vi "Edit Configrations.vi"(2 "Error In":errorcluster) -> (0 "Error Out":errorcluster)   [LabVIEW 2018]
uses:
  Type Defs/Instrument Model.ctl
  Type Defs/State Machine.ctl
  Config/Edit Config.ctl
  Type Defs/Configration.ctl
  GC-MSMSDevlopment/Type/_RT Configuration 2.ctl
  Type Defs/Global Action.ctl
  Type Defs/RT Command.ctl
  FGVs/Global Variables.vi
  <vilib>/Utility/config.llb/Read Key (Path).vi
  <vilib>/Utility/config.llb/Read Key (I32).vi
  <vilib>/Utility/config.llb/Read Key (Boolean).vi
  <vilib>/Utility/config.llb/Write Key (Path).vi
  <vilib>/Utility/config.llb/Write Key (String).vi
  <vilib>/Utility/config.llb/Write Key (Boolean).vi
  <vilib>/Utility/config.llb/Write Key (I32).vi
  <vilib>/Utility/config.llb/NI_LVConfig.lvlib
panel:
  in  "dsPIC33 4":u16
  in  "dsPIC33 3":u16
  in  "dsPIC33 2":u16
  in  "Set PIC":bool
  out "dsPIC33 Monitor":u64
  in  "dsPIC33":u16
  in  "Model Name":T1
  in  "Exit":bool
  in  "Pole Swap Options Negative":T2
  in  "Pole Swap Options Positive":T2
  in  "Dead Time":i32
  out "Number of Parameters":i32
  in  "CAD Evac T (ms)":i32
  in  "CAD Fill T (ms)":i32
  in  "S Swithc T (mS)":i32
  in  "Pole Swithc T (mS)":i32
  in  "Oscillator Settings":string[](array[string])
  in  "Restore From Power Failure":bool
  in  "Use DT Correction":bool
  in  "Enable Voltage Reset":bool
  in  "Serial Number":string
  in  "Config File Name":string
  in  "Settling Time (mS)":dbl
  in  "Description":string
  in  "Type":u8 format="%b"
  in  "Calibration Offset":dbl
  in  "Calibration Slop":dbl
  in  "User -ve Default":dbl
  in  "User +ve Default":dbl
  in  "User Maximum":dbl
  in  "User Minimum":dbl
  in  "Channel Number":u8
  in  "Parameter Name":string
  in  "Export":bool
  in  "Import":bool
  in  "Delete Row":bool
  in  "Insert Row":bool
  in  "Load":bool
  in  "Save":bool
  in  "Undo":bool
  in  "Reconnect":bool
  in  "Table":i32(listbox)
  # "Other Instrument Configrations"
  # "Pole Orientation"
  # "Current Parameters"
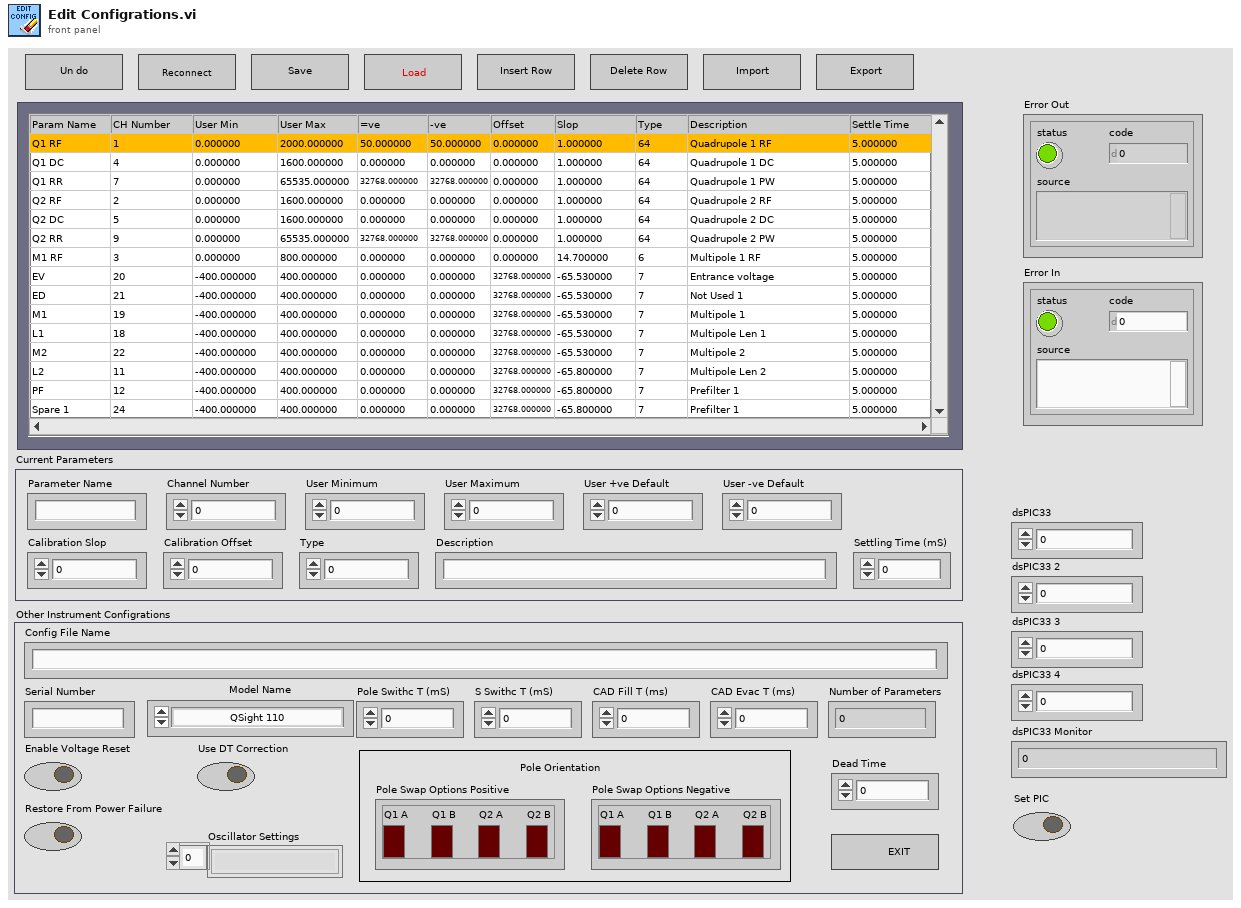
[diagram p1: front panel]
types:
  T1 = typedef "Instrument Model.ctl" = enum16{"QSight 110", "QSight 120", "QSight 210", "QSight 220", "QSight 410", "QSight 420", "IONICS 3Q 110", "IONICS 3Q 120", "IONICS 3Q 210", "IONICS 3Q 220", "IONICS 3Q 310", "IONICS 3Q 320", "Simulation (Single Source)", "Simulation (Dual Source)"}
  T2 = cluster{"Q1 A":bool, "Q1 B":bool, "Q2 A":bool, "Q2 B":bool}
  T3 = typedef "Edit Config.ctl" = cluster{"IP Address":string, "Index":i32, "Update Table":bool, "File Path":path, "Configration":T4}
  T4 = typedef "Configration.ctl" = cluster{"Table":T5[], "Instrument":string[]}
  T5 = typedef "_RT Configuration 2.ctl" = cluster{"Name":string, "Ch#":u8, "Min":dbl, "Max":dbl, "Def+":dbl, "Def-":dbl, "Offset":dbl, "Slope":dbl, "Type":u8, "Description":string, "SettleT":dbl}
  T6 = typedef "State Machine.ctl" = enum16{"Wait", "Init", "Case 0", "Case 1", "Case 2", "Case 3", "Case 4", "Case 5", "Case 6", "Case 7", "Case 8", "Case 9", "Case 10", "Error", "Exit"}
  T7 = typedef "Global Action.ctl" = enum16{"Write", "Read"}
  T8 = typedef "RT Command.ctl" = enum16{"xml Start Run", "xml Start Actual Run", "xml Stop Run", "xml Runtime Update", "xml Get Status", "xml Get Table", "xml Set Table", "xml Get Configuration", "xml System Status", "xml Set LC Input Logic", "xml Get Data", "xml Get Info", "Start", "StartActualRun", "Stop", "Runtime Update", "Get Data", "Get Info", "Get Status", "Get Param", "Get Config", "Get Table", "Read ADC", "Set Oscillator", "Update Config", "Update Table", "Set All Pol", "Set Pol and DC", "Set Max Mass", "Toggle RP", "Toggle EL", "Set PIC", "Initialize Turbo", "Send Turbo Comm", "Close Turbo", "P1", "P2", "P3", "Send Serial", "Set LC Out", "Get LC In", "Read VAC", "Test Table", "Toggle Power", "Get Startup", "Set Startup", "Get ADC Table", "Set ADC Table", "Get Brief Status", "Get Detail Status", "Auxiliary Update", "Set CC Logics", "Set CC Input Logics", "Ignore Error", "invalid"}
  T9 = typedef "Global Configrations.ctl" = cluster{"Model Name":enum16{"QSight 110", "QSight 120", "QSight 210", "QSight 220", "QSight 410", "QSight 420", "IONICS 3Q 110", "IONICS 3Q 120", "IONICS 3Q 210", "IONICS 3Q 220", "IONICS 3Q 310", "IONICS 3Q 320", "Simulation (Single Source)", "Simulation (Dual Source)"}, "RunType":u16, "Acquisition State":enum16{"Ready", "Busy", "Waiting"}, "InstrState":enum16{"Initializing", "Mass Spectrometer is Off", "Starting Up", "Turning Power Off", "Going to Standby", "Roughing Pump Ready", "Turning Turbo Off", "Turbo Startup", "Turbopump Ready", "Checking Vacuum", "Going to Ready", "Ready", "Running", "Source Standby", "Lost Communication", "Shutting Down", "Fault", "24V Standby", "Go to 24V Standby", "Turbopump Ready-Waiting"}, "Run Mode":enum16{"MRM (Q1/Q2)", "Q1 Scan", "Q1 SRM", "Q2 Scan", "Q2 SRM", "Product Scan", "Precursor Scan", "Neutral Loss", "Neutral Gain"}, "Configration":T4, "TCP ID":refnum<k5>, "DT":bool, "Dead Time (nS)":i32, "Single Source":bool, "ADC Tables":T10[], "FW Udate":bool, "Simulator":bool}
  T10 = typedef "ADC Table.ctl" = cluster{"Name":string, "Ch#":u8, "Min":dbl, "Max":dbl, "Def+":dbl, "Def-":dbl, "Offset":dbl, "Slope":dbl, "Type":u8, "Description":string, "SettleT":dbl}
  T11 = typedef "NI_LVConfig.lvlib/Config Data RefNum.ctl" = refnum<k1>
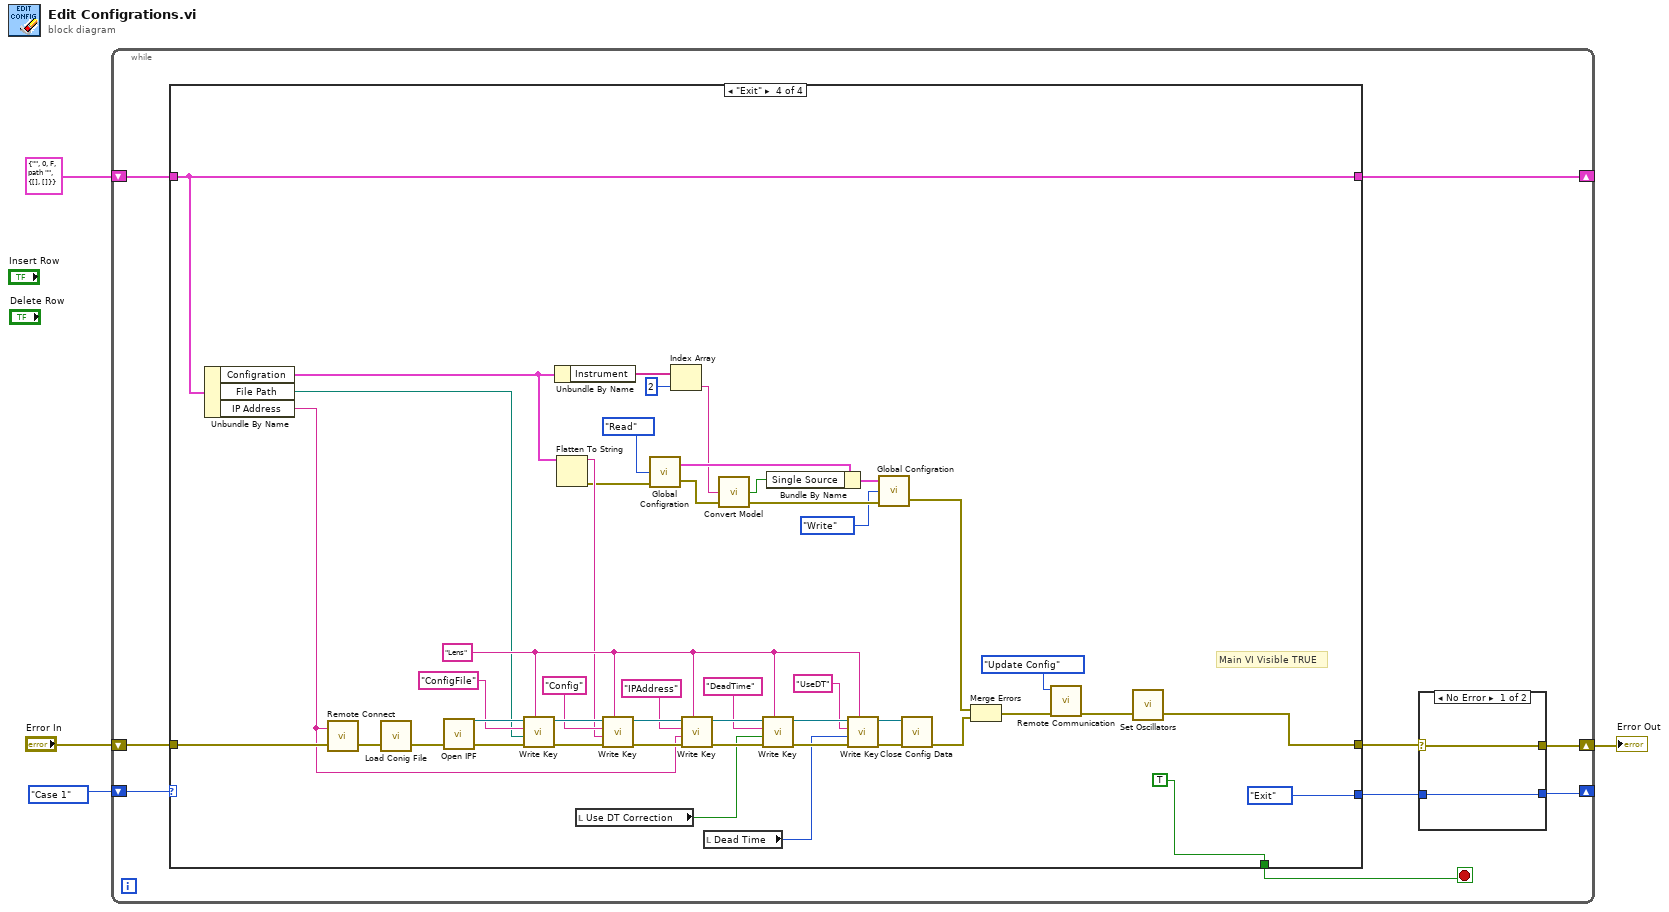
[diagram p0: block diagram]
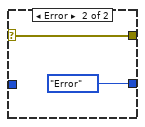
[diagram p2: hidden frame]
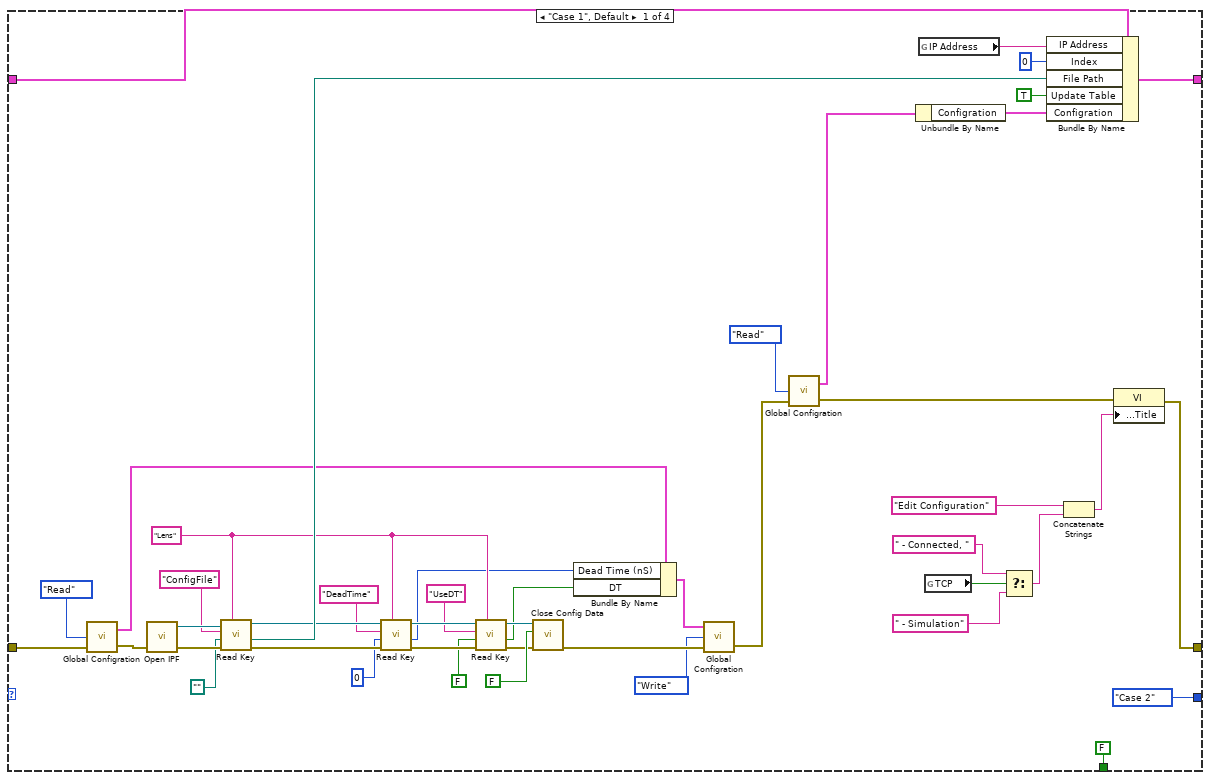
[diagram p3: hidden frame]
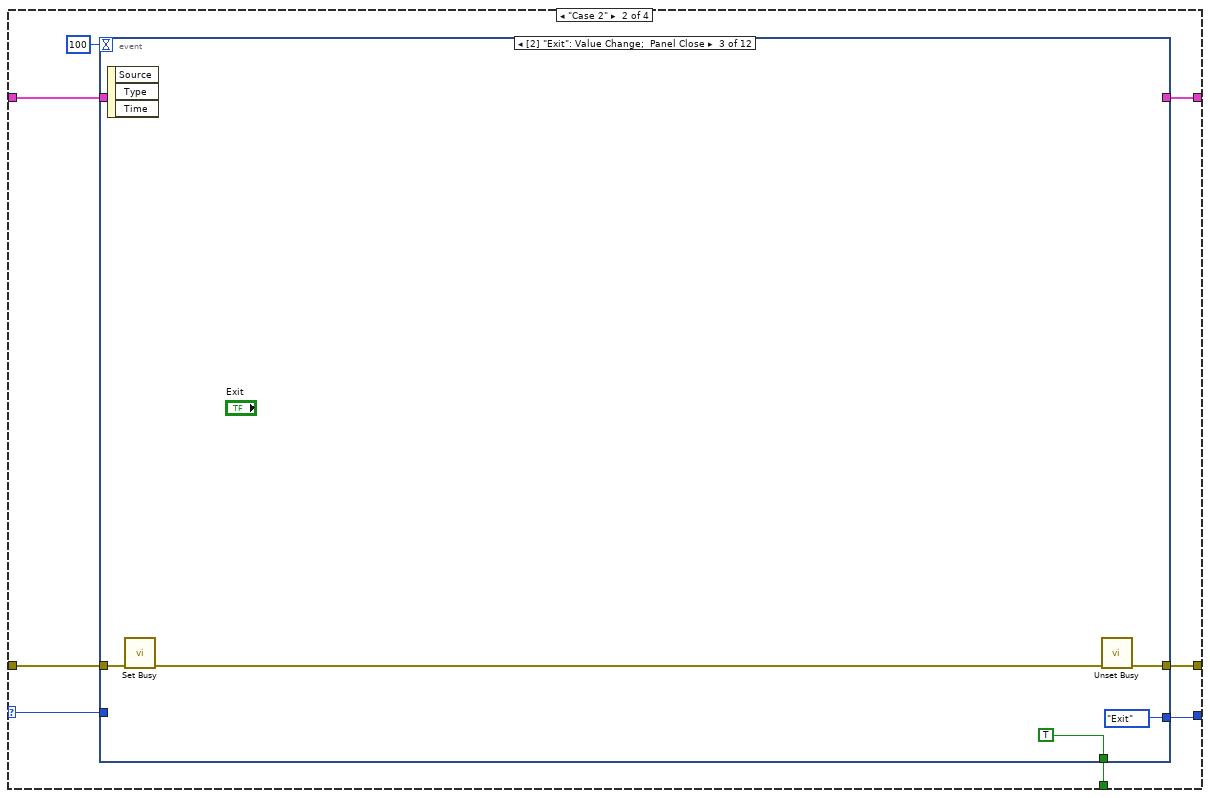
[diagram p4: hidden frame]
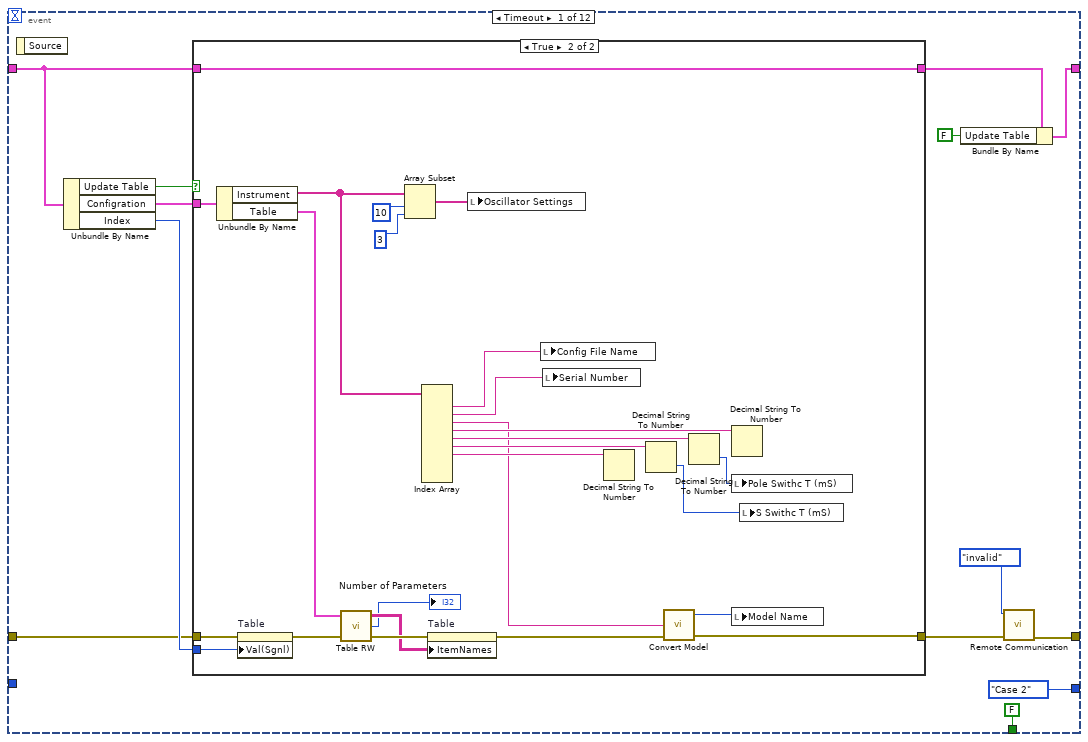
[diagram p5: hidden frame]
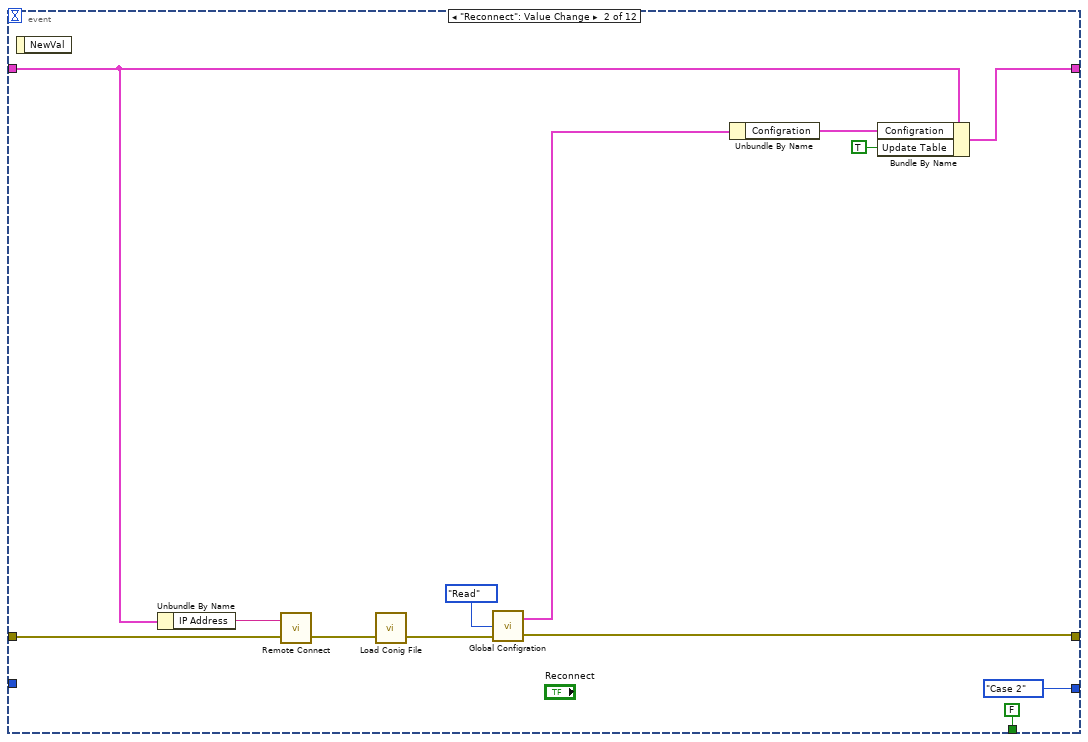
[diagram p7: hidden frame]
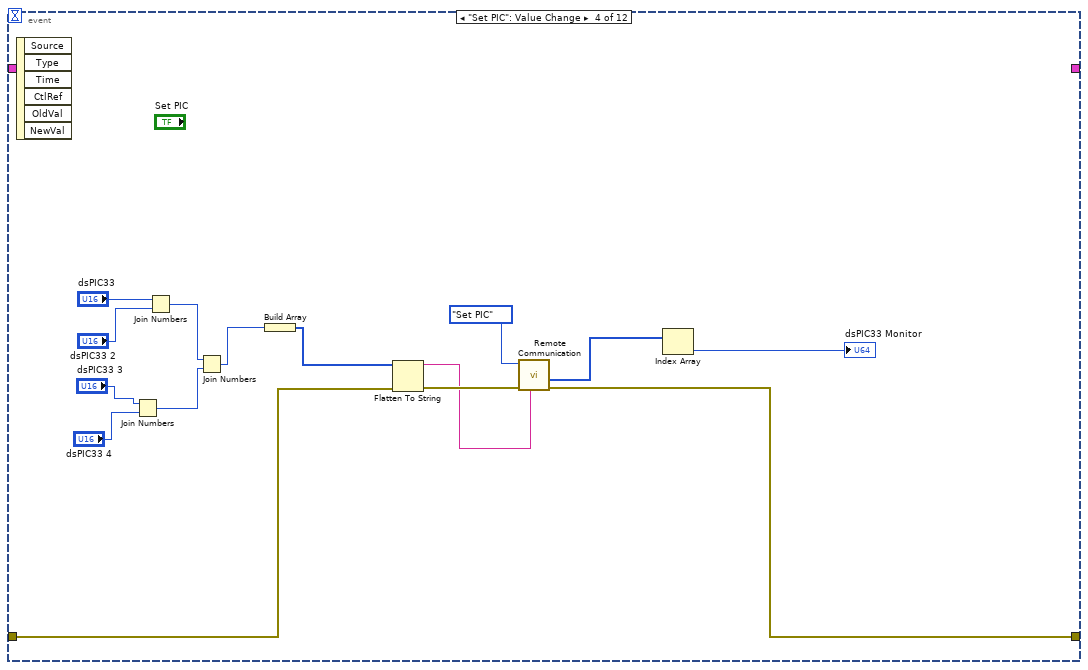
[diagram p8: hidden frame]
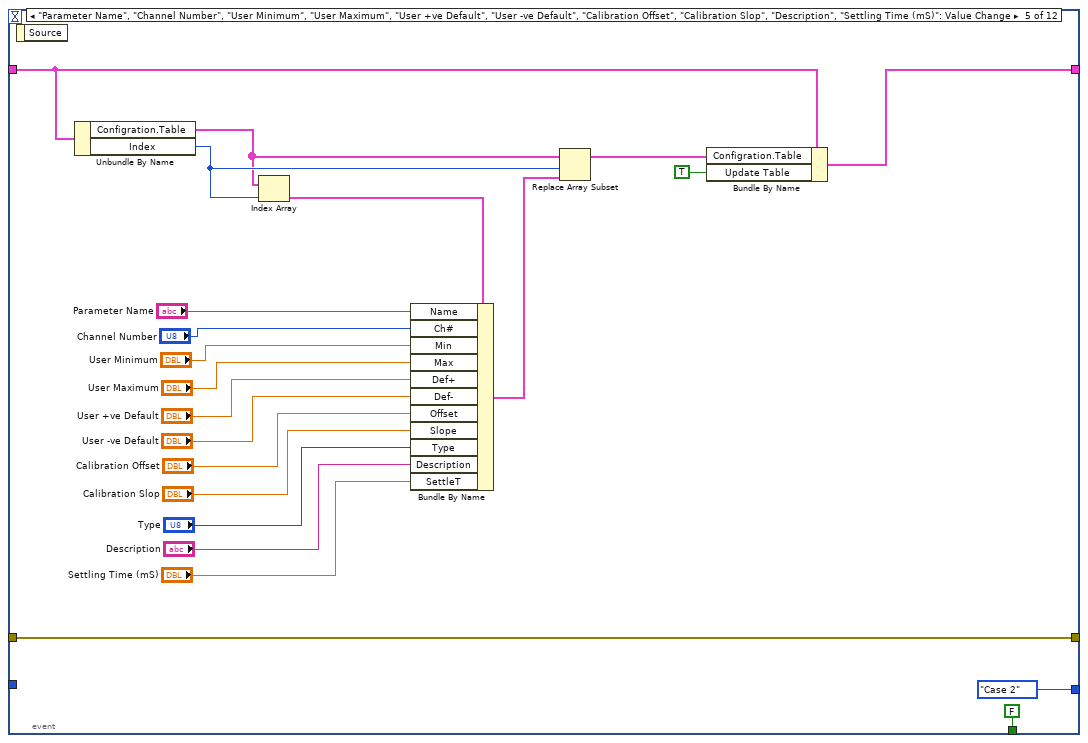
[diagram p9: hidden frame]
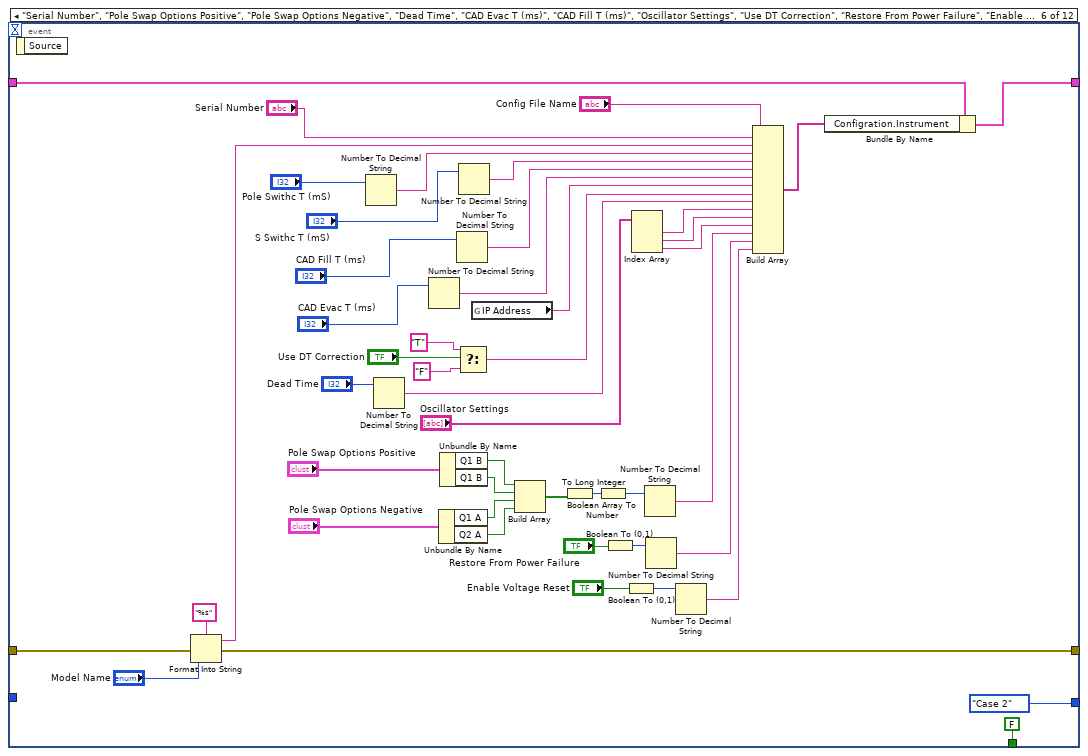
[diagram p10: hidden frame]
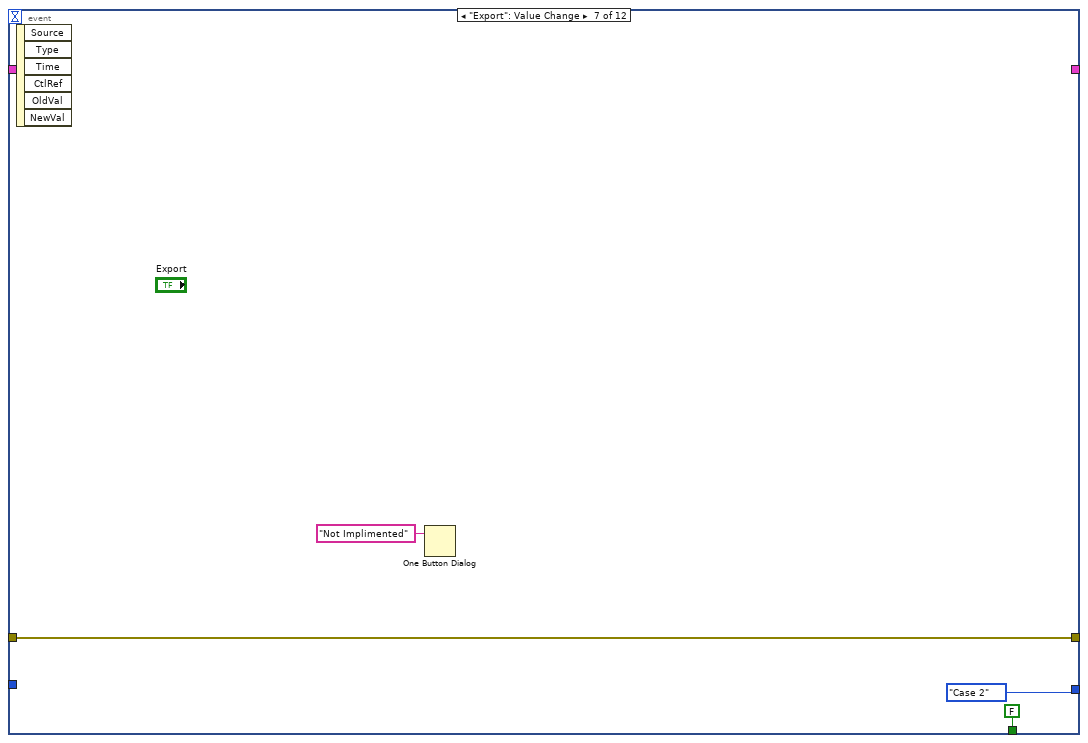
[diagram p11: hidden frame]
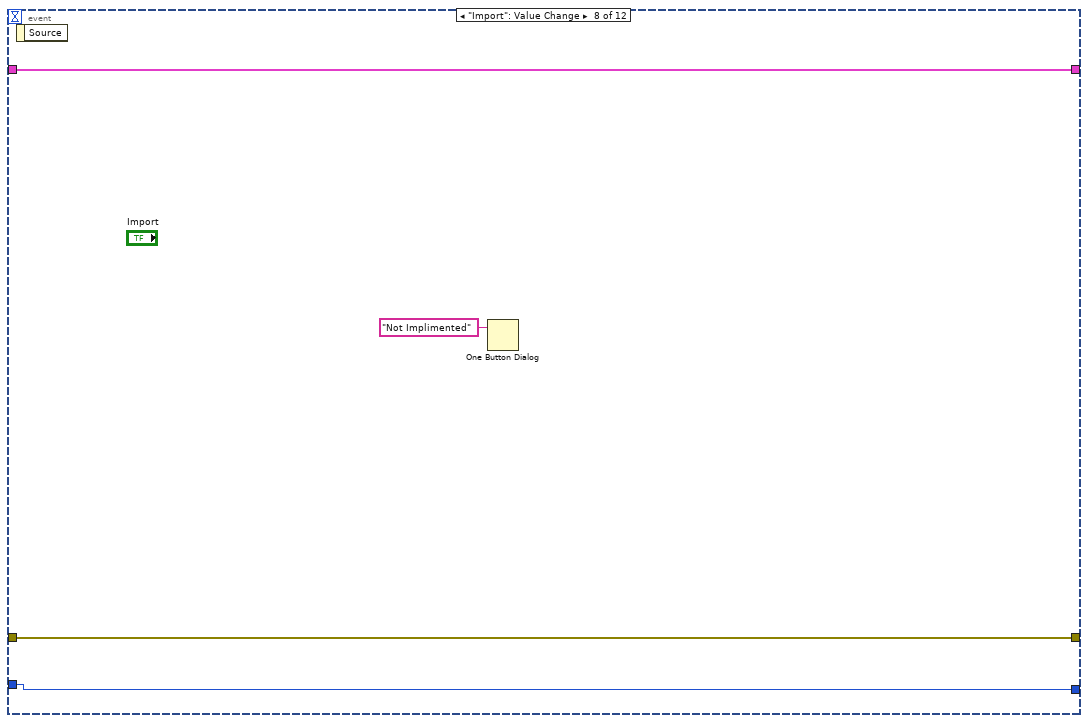
[diagram p12: hidden frame]
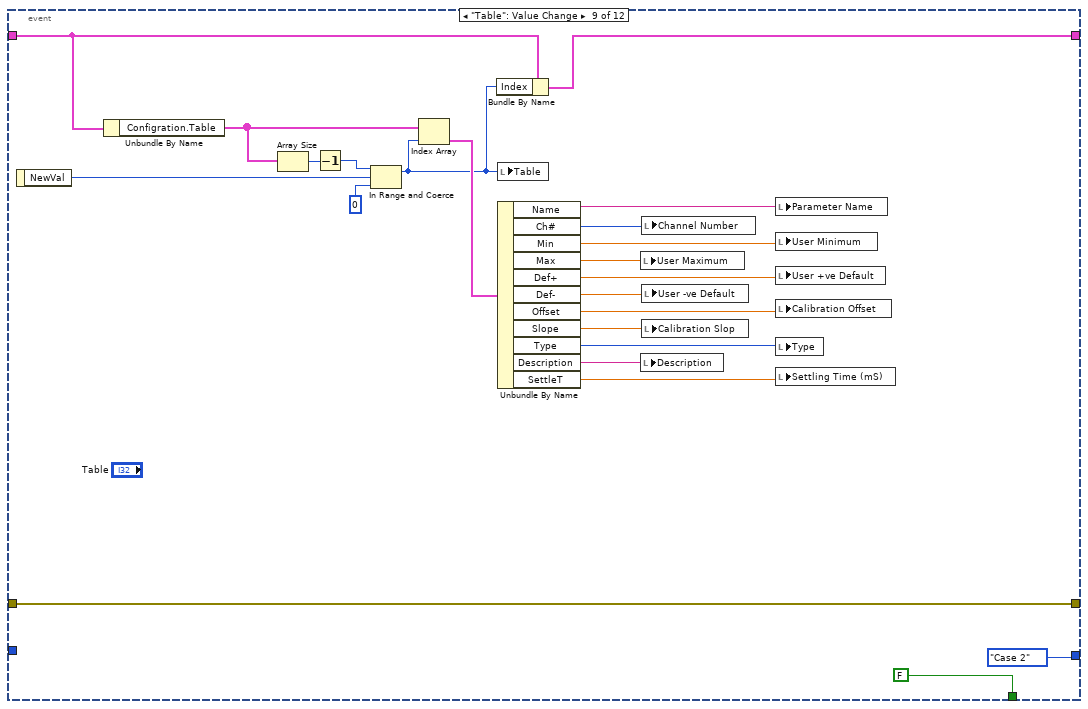
[diagram p13: hidden frame]
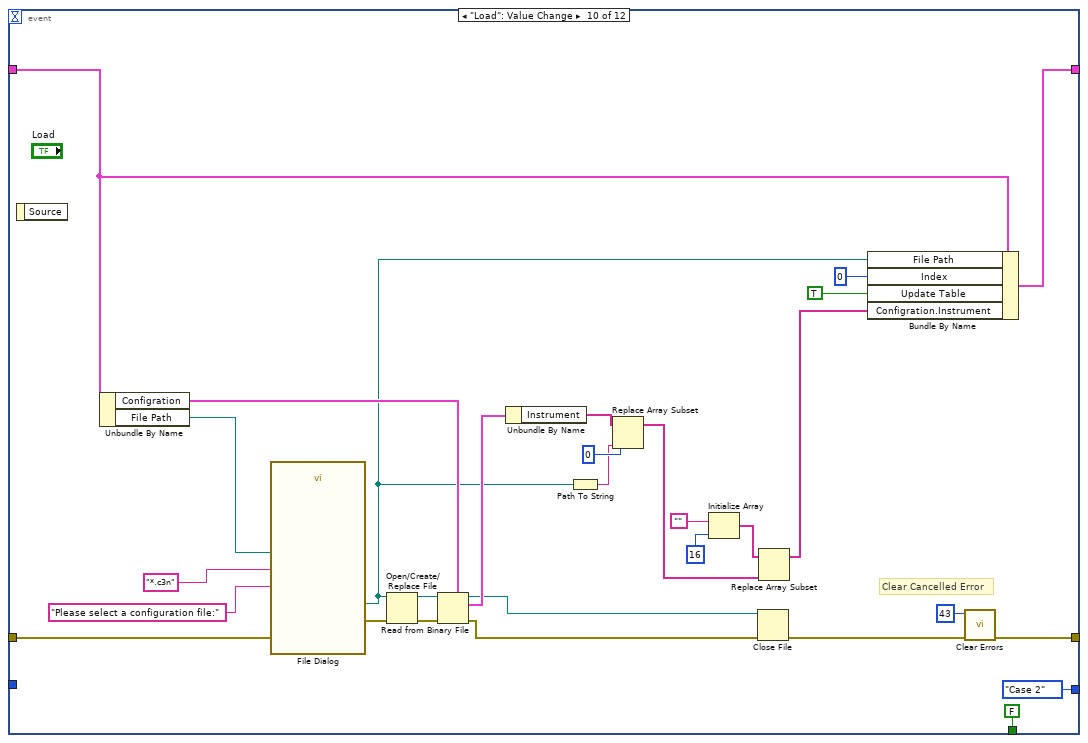
[diagram p14: hidden frame]
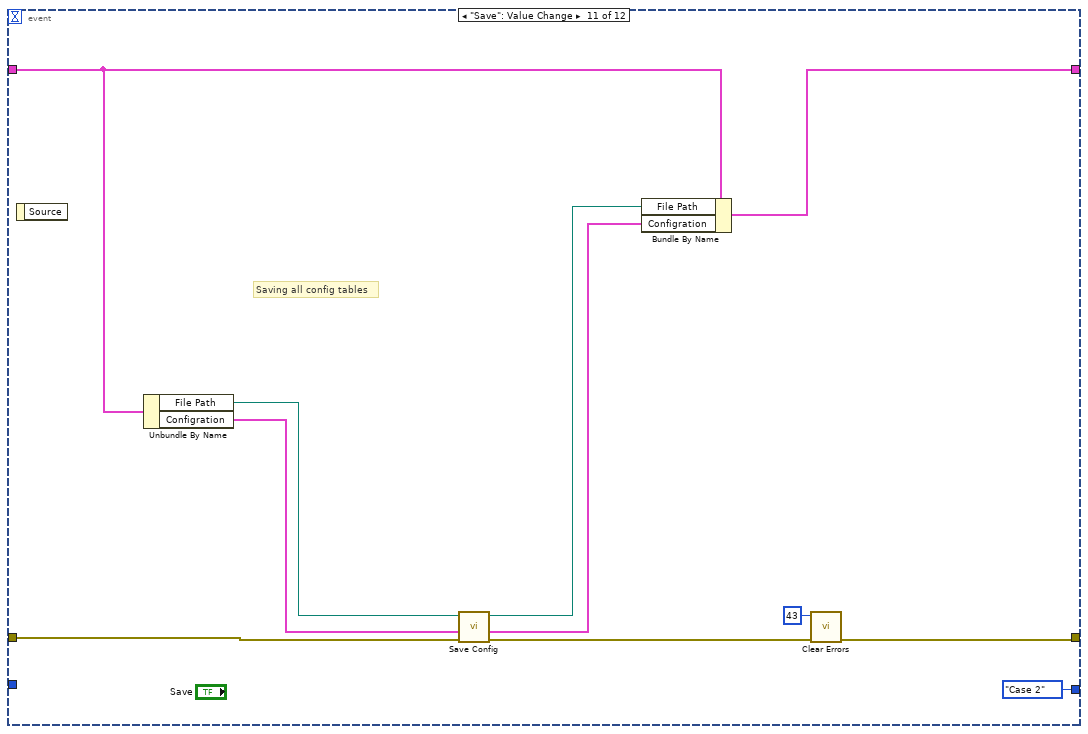
[diagram p15: hidden frame]
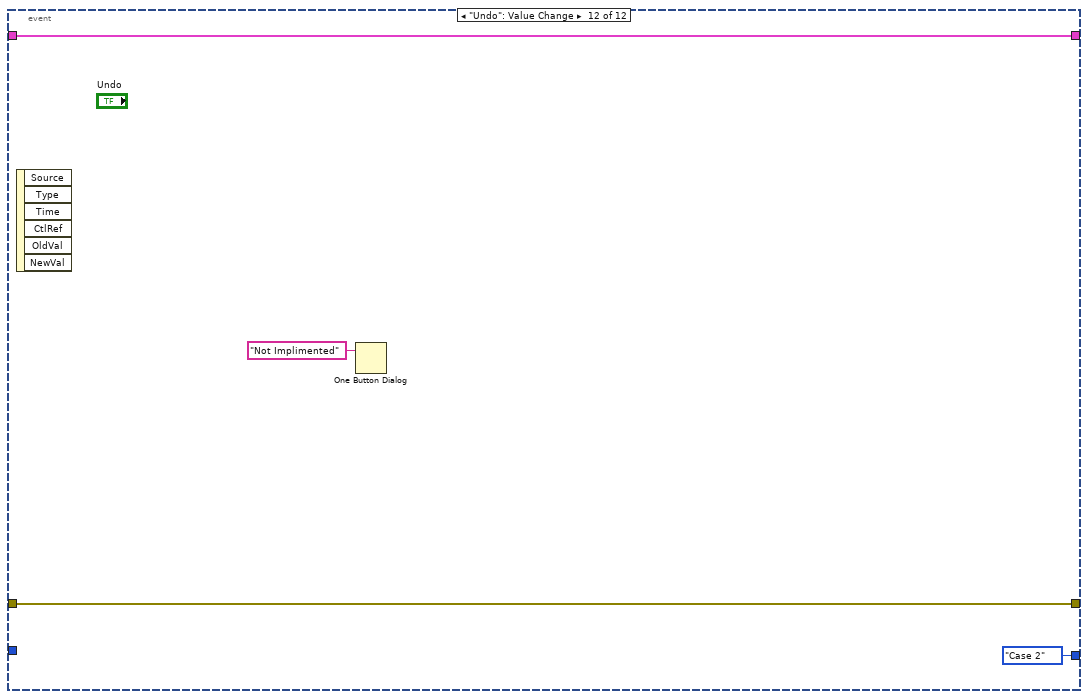
[diagram p16: hidden frame]
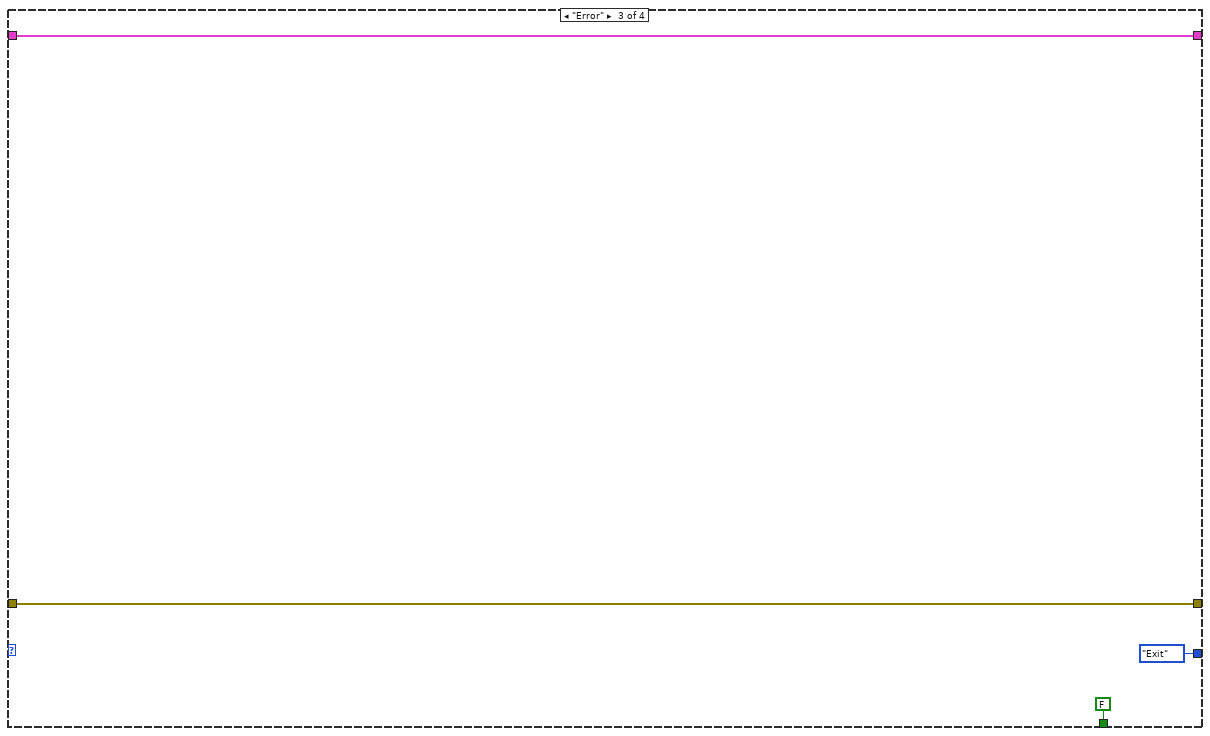
[diagram p17: hidden frame]
diagram:
  n1 = while {
    shift-right: [w8] -> _
    shift-left: State_Machine."Case 1" -> [w13]
    shift-right: [w11] -> _
    shift-left: T3 {"IP Address"="", "Index"=0, "Update Table"=FALSE, "File Path"=path "", "Configration"={"Table"=[], "Instrument"=[]}} ("Edit Configrations") -> [w10]
    shift-right: [w6] -> w2
    shift-left: "Error In" -> [w12]
    stop <- w5 stop-if-true
    n2 = case shown="\"Exit\"" w13 {
      selector: w13 -> [_ w66 _ _]
      tunnel: w12 -> [w27 w69 w288 w313]
      tunnel: [w62 w67 w289 w337] -> w11
      tunnel: [w50 w68 w288 w292] -> w9
      tunnel: w10 -> [w24 w70 w289 w337]
      tunnel: [State_Machine."Case 2" w64 State_Machine."Exit" State_Machine."Exit"] -> w7
      tunnel: [FALSE w63 FALSE TRUE] -> w5
      frame "Case 1", Default {
        w40 = "Lens" ("section")
        n3 = call "Global Configration.vi"("Error In"=w27, "Action"=Global_Action."Read") -> ("Error Out"=w28:errorcluster, "Parameters Out"=w25:T9)  [unwired: 1 in]
        n4 = call "Open IPF.vi"("Error In"=w28) -> ("Error Out"=w57:errorcluster, "IPF refnum"=w56:T11)  [unwired: 2 in, 1 out]
        n5 = call-poly <vilib>:"Read Key.vi"("section"=w40, "error in (no error)"=w57, "default value"=path "", "key"="ConfigFile", "refnum"=w56) -> ("error out"=w52:errorcluster, "value"=w53:path, "refnum out"=w51:T11)  [unwired: 4 out]
        n6 = call-poly <vilib>:"Read Key.vi"("section"=w40, "error in (no error)"=w52, "default value"=0, "key"="DeadTime", "refnum"=w51) -> ("error out"=w43:errorcluster, "value"=w31:i32, "refnum out"=w41:T11)  [unwired: 4 out]
        n7 = call-poly <vilib>:"Read Key.vi"("section"=w40, "error in (no error)"=w43, "default value"=FALSE, "key"="UseDT", "refnum"=w41) -> ("error out"=w34:errorcluster, "value"=w32:bool, "refnum out"=w42:T11)  [unwired: 4 out]
        n8 = call <vilib>:"Close Config Data.vi"("error in (no error)"=w34, "write file if changed (T)"=FALSE, "refnum"=w42) -> ("error out"=w30:errorcluster)  [unwired: 8 out]
        n9 = Bundle By Name(cluster=w25, "Dead Time (nS)"=w31, "DT"=w32) -> (w33:T9)
        n10 = call "Global Configration.vi"("Error In"=w30, "Action"=Global_Action."Write", "Parameters In"=w33) -> ("Error Out"=w20:errorcluster)  [unwired: 1 out]
        n11 = call "Global Configration.vi"("Error In"=w20, "Action"=Global_Action."Read") -> ("Error Out"=w21:errorcluster, "Parameters Out"=w19:T9)  [unwired: 1 in]
        n12 = Unbundle By Name(w19) -> ("Configration"=w58:T4)
        n13 = global read "Global Variables.vi" "IP Address"() -> (w61:string)
        n14 = global read "Global Variables.vi" "TCP"() -> (w46:bool)
        n15 = Select(t=" - Connected, " ("string"), s=w46, f=" - Simulation" ("string")) -> (s? t:f=w47:string)
        n16 = Bundle By Name(cluster=w24, "IP Address"=w61, "Index"=0, "File Path"=w53, "Update Table"=TRUE, "Configration"=w58) -> (w62:T3)
        n17 = Concatenate Strings("Edit Configuration" ("string"), w47) -> (w44:string)
        n18 = property class="VI"(error in=w21, "Front Panel Window:Title"=w44) -> (error out=w50:errorcluster)  [unwired: 1 in, 1 out]
      }
      frame "Case 2" {
        n19 = event shown="[2] \"Exit\": Value Change;  Panel Close" {
          selector: _ -> [_ _ _ _ _ _ _ _ _ _ _ _]
          dyn-events: _ -> [_ _ _ _ _ _ _ _ _ _ _ _]
          timeout: 100 -> [_ _ _ _ _ _ _ _ _ _ _ _]
          tunnel: w70 -> [w76 w119 _ _ w161 w212 _ w219 w235 w263 w280 w286]
          tunnel: [FALSE FALSE TRUE _ FALSE FALSE FALSE _ FALSE FALSE _ _] -> w63
          tunnel: w69 -> [w78 w123 w126 w141 w146 w205 w215 w218 w242 w270 w283 w285]
          tunnel: [w73 w113 w125 w138 w146 w203 w215 w218 w242 w244 w274 w285] -> w68
          tunnel: [w83 w118 _ _ w158 w211 _ w219 w234 w249 w277 w286] -> w67
          tunnel: w66 -> [_ _ _ _ _ _ _ w217 _ _ _ _]
          tunnel: [State_Machine."Case 2" State_Machine."Case 2" State_Machine."Exit" _ State_Machine."Case 2" State_Machine."Case 2" State_Machine."Case 2" w217 State_Machine."Case 2" State_Machine."Case 2" State_Machine."Case 2" State_Machine."Case 2"] -> w64
          event Timeout {
            n20 = event-data() -> ()  [unwired: 1 in, 1 out]
            n21 = Unbundle By Name(w76) -> ("Update Table"=w81:bool, "Configration"=w80:T4, "Index"=w79:i32)
            n22 = case shown="True" w81 {
              tunnel: w80 -> [_ w110]
              tunnel: w79 -> [_ w108]
              tunnel: w78 -> [w85 w109]
              tunnel: [w85 w90] -> w72
              tunnel: [w84 w86] -> w75
              tunnel: w76 -> [w84 w86]
              frame False {
              }
              frame True {
                n23 = Unbundle By Name(w110) -> ("Instrument"=w88:string[], "Table"=w106:T5[])
                n24 = property on="Table" class="MCListbox (strict)"(error in=w109, "Val(Sgnl)"=w108) -> (error out=w107:errorcluster)  [unwired: 1 in, 1 out]
                n25 = call "Table RW.vi"("Error In"=w107, "Table In"=w106) -> ("Error Out"=w105:errorcluster, "Number of param"=→"Number of Parameters":i32, "List Out"=w104:string[][])  [unwired: 1 in]
                n26 = Array Subset(array=w88, index=10, length=3) -> (w99:string[])
                n27 = Index Array(array=w88) -> (element #1=w103:string, element #2=w102:string, element #3=w89:string, element #4=w98:string, element #5=w97:string, element #6=w96:string, element #7=w95:string)  [unwired: 10 in, 3 out]
                n28 = property on="Table" class="MCListbox (strict)"(error in=w105, "ItemNames"=w104) -> (error out=w91:errorcluster)  [unwired: 1 in, 1 out]
                n29 = local write "Oscillator Settings"(w99) -> ()
                n30 = local write "Config File Name"(w103) -> ()
                n31 = local write "Serial Number"(w102) -> ()
                n32 = Decimal String To Number(string=w95) -> ()  [unwired: 4 out]
                n33 = Decimal String To Number(string=w96) -> (number=w93:i32)  [unwired: 3 out]
                n34 = call "Convert Model.vi"("error in (no error)"=w91, "Model"=w89) -> ("error out"=w90:errorcluster, "Model Name  Out"=w87:T1)  [unwired: 1 in, 1 out]
                n35 = Decimal String To Number(string=w97) -> (number=w94:i32)  [unwired: 3 out]
                n36 = Decimal String To Number(string=w98) -> ()  [unwired: 4 out]
                n37 = local write "Pole Swithc T (mS)"(w94) -> ()
                n38 = local write "Model Name"(w87) -> ()
                n39 = local write "S Swithc T (mS)"(w93) -> ()
              }
            }
            n40 = Bundle By Name(cluster=w75, "Update Table"=FALSE) -> (w83:T3)
            n41 = call "Remote Communication.vi"("Error In"=w72, "Command"=RT_Command."invalid") -> ("Error Out"=w73:errorcluster)  [unwired: 4 in, 3 out]
          }
          event "Reconnect": Value Change {
            n42 = event-data() -> ()  [unwired: 1 in, 1 out]
            n43 = Unbundle By Name(w119) -> ("IP Address"=w122:string)
            n44 = call "Remote Connect.vi"("Error In"=w123, "IP Address"=w122) -> ("Error Out"=w121:errorcluster)  [unwired: 1 out]
            n45 = call "Load Conig File.vi"("error in (no error)"=w121) -> ("error out"=w117:errorcluster)  [unwired: 1 in, 1 out]
            n46 = call "Global Configration.vi"("Error In"=w117, "Action"=Global_Action."Read") -> ("Error Out"=w113:errorcluster, "Parameters Out"=w115:T9)  [unwired: 1 in]
            n47 = Unbundle By Name(w115) -> ("Configration"=w114:T4)
            n48 = Bundle By Name(cluster=w119, "Configration"=w114, "Update Table"=TRUE) -> (w118:T3)
          }
          event "Exit": Value Change; Panel Close {
            n49 = event-data() -> ()  [unwired: 1 in, 3 out]
            n50 = call <vilib>:"Set Busy.vi"("error in (no error)"=w126) -> ("error out"=w124:errorcluster)  [unwired: 9 in, 1 out]
            n51 = call <vilib>:"Unset Busy.vi"("error in (no error)"=w124) -> ("error out"=w125:errorcluster)  [unwired: 10 in]
          }
          event "Set PIC": Value Change {
            n52 = event-data() -> ()  [unwired: 1 in, 6 out]
            n53 = Join Numbers(hi="dsPIC33 3", lo="dsPIC33 4") -> ((hi.lo)=w129:u32)
            n54 = Join Numbers(hi="dsPIC33", lo="dsPIC33 2") -> ((hi.lo)=w130:u32)
            n55 = Join Numbers(hi=w130, lo=w129) -> ((hi.lo)=w131:u64)
            n56 = Build Array(w131) -> (w142:u64[])
            n57 = Flatten To String(anything=w142, error in (no error)=w141) -> (data string=w140:string, error out=w143:errorcluster)  [unwired: 3 out]
            n58 = call "Remote Communication.vi"("String"=w140, "Error In"=w143, "Command"=RT_Command."Set PIC") -> ("Error Out"=w138:errorcluster, "Data Array"=w134:i32[])  [unwired: 3 in, 2 out]
            n59 = Index Array(array=w134) -> (element=→"dsPIC33 Monitor":i32)  [unwired: 1 in]
          }
          event "Parameter Name", "Channel Number", "User Minimum", "User Maximum", "User +ve Default", "User -ve Default", "Calibration Offset", "Calibration Slop", "Description", "Settling Time (mS)": Value Change {
            n60 = event-data() -> ()  [unwired: 1 in, 1 out]
            n61 = Unbundle By Name(w161) -> ("Configration.Table"=w163:T5[], "Index"=w164:i32)
            n62 = Index Array(array=w163, index=w164) -> (element=w165:T5)
            n63 = Bundle By Name(cluster=w165, "Name"="Parameter Name", "Ch#"="Channel Number", "Min"="User Minimum", "Max"="User Maximum", "Def+"="User +ve Default", "Def-"="User -ve Default", "Offset"="Calibration Offset", "Slope"="Calibration Slop", "Type"="Type", "Description"="Description", "SettleT"="Settling Time (mS)") -> (w162:T5)
            n64 = Replace Array Subset(array=w163, new element=w162, index=w164) -> (w160:T5[])
            n65 = Bundle By Name(cluster=w161, "Configration.Table"=w160, "Update Table"=TRUE) -> (w158:T3)
          }
          event "Serial Number", "Pole Swap Options Positive", "Pole Swap Options Negative", "Dead Time", "CAD Evac T (ms)", "CAD Fill T (ms)", "Oscillator Settings", "Use DT Correction", "Restore From Power Failure", "Enable Voltage Reset": Value Change {
            n66 = event-data() -> ()  [unwired: 1 in, 1 out]
            n67 = Format Into String(format string="%s", error in=w205, "Model Name") -> (resulting string=w204:string, error out=w203:errorcluster)  [unwired: 1 in]
            n68 = Number To Decimal String(number="Pole Swithc T (mS)") -> (decimal integer string=w201:string)  [unwired: 1 out]
            n69 = Number To Decimal String(number="Dead Time") -> (decimal integer string=w188:string)  [unwired: 1 out]
            n70 = Number To Decimal String(number="CAD Evac T (ms)") -> (decimal integer string=w197:string)  [unwired: 1 out]
            n71 = Unbundle By Name("Pole Swap Options Negative") -> ("Q1 A"=w183:bool, "Q2 A"=w182:bool)
            n72 = Unbundle By Name("Pole Swap Options Positive") -> ("Q1 B"=w185:bool, "Q1 B"=w184:bool)
            n73 = Number To Decimal String(number="CAD Fill T (ms)") -> (decimal integer string=w198:string)  [unwired: 1 out]
            n74 = Select(t="T", s="Use DT Correction", f="F") -> (s? t:f=w192:string)
            n75 = Number To Decimal String(number="S Swithc T (mS)") -> (decimal integer string=w199:string)  [unwired: 1 out]
            n76 = global read "Global Variables.vi" "IP Address"() -> (w194:string)
            n77 = Build Array(w185, w184, w183, w182) -> (w179:bool[])
            n78 = Boolean Array To Number(Boolean array=w179) -> (number=w181:u32)
            n79 = To Long Integer(number=w181) -> (32bit integer=w180:i32)
            n80 = Boolean To (0,1)(Boolean="Restore From Power Failure") -> (0, 1=w172:i16)
            n81 = Boolean To (0,1)(Boolean="Enable Voltage Reset") -> (0, 1=w170:i16)
            n82 = Index Array(array="Oscillator Settings") -> (element #1=w177:string, element #2=w176:string, element #3=w175:string)  [unwired: 3 in]
            n83 = Number To Decimal String(number=w180) -> (decimal integer string=w174:string)  [unwired: 1 out]
            n84 = Number To Decimal String(number=w172) -> (decimal integer string=w169:string)  [unwired: 1 out]
            n85 = Number To Decimal String(number=w170) -> (decimal integer string=w168:string)  [unwired: 1 out]
            n86 = Build Array("Config File Name", "Serial Number", w204, w201, w199, w198, w197, w194, w192, w188, w177, w176, w175, w174, w169, w168) -> (w210:string[])
            n87 = Bundle By Name(cluster=w212, "Configration.Instrument"=w210) -> (w211:T3)
          }
          event "Export": Value Change {
            n88 = event-data() -> ()  [unwired: 1 in, 6 out]
            n89 = One Button Dialog(message="Not Implimented") -> ()  [unwired: 1 in, 1 out]
          }
          event "Import": Value Change {
            n90 = event-data() -> ()  [unwired: 1 in, 1 out]
            n91 = One Button Dialog(message="Not Implimented") -> ()  [unwired: 1 in, 1 out]
          }
          event "Table": Value Change {
            n92 = event-data() -> ("NewVal"=w236:i32)  [unwired: 1 in]
            n93 = Unbundle By Name(w235) -> ("Configration.Table"=w237:T5[])
            n94 = Array Size(array=w237) -> (size(s)=w240:i32)
            n95 = Decrement(x=w240) -> (x-1=w238:i32)
            n96 = In Range and Coerce(upper limit=w238, x=w236, lower limit=0) -> (coerced(x)=w233:i32)  [unwired: 1 out]
            n97 = Index Array(array=w237, index=w233) -> (element=w241:T5)
            n98 = Bundle By Name(cluster=w235, "Index"=w233) -> (w234:T3)
            n99 = local write "Table"(w233) -> ()
            n100 = Unbundle By Name(w241) -> ("Name"=w226:string, "Ch#"=w230:u8, "Min"=w224:dbl, "Max"=w225:dbl, "Def+"=w223:dbl, "Def-"=w222:dbl, "Offset"=w221:dbl, "Slope"=w227:dbl, "Type"=w228:u8, "Description"=w232:string, "SettleT"=w229:dbl)
            n101 = local write "User Maximum"(w225) -> ()
            n102 = local write "Description"(w232) -> ()
            n103 = local write "Channel Number"(w230) -> ()
            n104 = local write "User -ve Default"(w222) -> ()
            n105 = local write "Calibration Slop"(w227) -> ()
            n106 = local write "Parameter Name"(w226) -> ()
            n107 = local write "User Minimum"(w224) -> ()
            n108 = local write "User +ve Default"(w223) -> ()
            n109 = local write "Calibration Offset"(w221) -> ()
            n110 = local write "Type"(w228) -> ()
            n111 = local write "Settling Time (mS)"(w229) -> ()
          }
          event "Load": Value Change {
            # "Clear Cancelled Error"
            n112 = event-data() -> ()  [unwired: 1 in, 1 out]
            n113 = Unbundle By Name(w263) -> ("Configration"=w262:T4, "File Path"=w267:path)
            n114 = call "File Dialog"("start path"=w267, "prompt"="Please select a configuration file:", "error in"=w270, "pattern (all files)"="*.c3n" ("pattern (*.cfg)")) -> ("selected path"=w253:path, "error out"=w266:errorcluster)  [unwired: 8 in, 2 out]
            n115 = Open/Create/Replace File(file path (use dialog)=w253, error in=w266) -> (refnum out=w264:refnum<file>, error out=w265:errorcluster)  [unwired: 4 in, 1 out]
            n116 = Read from Binary File(5:w262, 8:w265, 11:w264) -> (0:w248:errorcluster, 2:w254:T4, 3:w247:refnum<file>)  [unwired: 4 out]
            n117 = Unbundle By Name(w254) -> ("Instrument"=w261:string[])
            n118 = Path To String(path=w253) -> (string=w259:string)
            n119 = Replace Array Subset(array=w261, new element=w259, index=0) -> (w255:string[])
            n120 = Initialize Array("", 16 ("dimension size")) -> (w258:string[])
            n121 = Close File(refnum=w247, error in=w248) -> (error out=w245:errorcluster)  [unwired: 1 out]
            n122 = Replace Array Subset(array=w258, new element=w255) -> (w250:string[])  [unwired: 1 in]
            n123 = Bundle By Name(cluster=w263, "File Path"=w253, "Index"=0, "Update Table"=TRUE, "Configration.Instrument"=w250) -> (w249:T3)
            n124 = call <vilib>:"Clear Errors.vi"("error in (no error)"=w245, "specific error code to clear (0: all)"=43) -> ("error out"=w244:errorcluster)  [unwired: 4 in, 1 out]
          }
          event "Save": Value Change {
            # "Saving all config tables"
            n125 = event-data() -> ()  [unwired: 1 in, 1 out]
            n126 = Unbundle By Name(w280) -> ("File Path"=w281:path, "Configration"=w282:T4)
            n127 = call "Save Config.vi"("Error In"=w283, "Configuration In"=w282, "File Path In"=w281) -> ("Error Out"=w275:errorcluster, "Configration Out"=w279:T4, "File Path Out"=w278:path)  [unwired: 1 in, 1 out]
            n128 = Bundle By Name(cluster=w280, "File Path"=w278, "Configration"=w279) -> (w277:T3)
            n129 = call <vilib>:"Clear Errors.vi"("error in (no error)"=w275, "specific error code to clear (0: all)"=43) -> ("error out"=w274:errorcluster)  [unwired: 4 in, 1 out]
          }
          event "Undo": Value Change {
            n130 = event-data() -> ()  [unwired: 1 in, 6 out]
            n131 = One Button Dialog(message="Not Implimented") -> ()  [unwired: 1 in, 1 out]
          }
        }
      }
      frame "Error" {
      }
      frame "Exit" {
        w324 = "Lens" ("section")
        # "Main VI Visible TRUE"
        n132 = Unbundle By Name(w337) -> ("Configration"=w310:T4, "File Path"=w317:path, "IP Address"=w297:string)
        n133 = call "Remote Connect.vi"("Error In"=w313, "IP Address"=w297) -> ("Error Out"=w336:errorcluster)  [unwired: 1 out]
        n134 = call "Load Conig File.vi"("error in (no error)"=w336) -> ("error out"=w335:errorcluster)  [unwired: 1 in, 1 out]
        n135 = call "Open IPF.vi"("Error In"=w335) -> ("Error Out"=w334:errorcluster, "IPF refnum"=w333:T11)  [unwired: 2 in, 1 out]
        n136 = call-poly <vilib>:"Write Key.vi"("section"=w324, "error in (no error)"=w334, "value"=w317, "key"="ConfigFile", "refnum"=w333) -> ("error out"=w332:errorcluster, "refnum out"=w328:T11)  [unwired: 5 out]
        n137 = Unbundle By Name(w310) -> ("Instrument"=w309:string[])
        n138 = Flatten To String(anything=w310) -> (data string=w318:string, error out=w312:errorcluster)  [unwired: 1 in, 3 out]
        n139 = local read "Use DT Correction"() -> (w296:bool)
        n140 = call-poly <vilib>:"Write Key.vi"("section"=w324, "error in (no error)"=w332, "value"=w318, "key"="Config" ("section"), "refnum"=w328) -> ("error out"=w331:errorcluster, "refnum out"=w327:T11)  [unwired: 1 in, 4 out]
        n141 = call "Global Configration.vi"("Error In"=w312, "Action"=Global_Action."Read") -> ("Error Out"=w306:errorcluster, "Parameters Out"=w308:T9)  [unwired: 1 in]
        n142 = Index Array(array=w309, index=2) -> (element=w307:string)
        n143 = call-poly <vilib>:"Write Key.vi"("section"=w324, "error in (no error)"=w331, "value"=w297, "key"="IPAddress" ("section"), "refnum"=w327) -> ("error out"=w330:errorcluster, "refnum out"=w326:T11)  [unwired: 1 in, 4 out]
        n144 = local read "Dead Time"() -> (w295:i32)
        n145 = call "Convert Model.vi"("error in (no error)"=w306, "Model"=w307) -> ("error out"=w304:errorcluster, "SingleSource"=w305:bool)  [unwired: 1 in, 1 out]
        n146 = call-poly <vilib>:"Write Key.vi"("section"=w324, "error in (no error)"=w330, "value"=w296, "key"="DeadTime", "refnum"=w326) -> ("error out"=w329:errorcluster, "refnum out"=w325:T11)  [unwired: 5 out]
        n147 = Bundle By Name(cluster=w308, "Single Source"=w305) -> (w303:T9)
        n148 = call-poly <vilib>:"Write Key.vi"("section"=w324, "error in (no error)"=w329, "value"=w295, "key"="UseDT", "refnum"=w325) -> ("error out"=w316:errorcluster, "refnum out"=w315:T11)  [unwired: 5 out]
        n149 = call "Global Configration.vi"("Error In"=w304, "Action"=Global_Action."Write", "Parameters In"=w303) -> ("Error Out"=w301:errorcluster)  [unwired: 1 out]
        n150 = call <vilib>:"Close Config Data.vi"("error in (no error)"=w316, "refnum"=w315) -> ("error out"=w302:errorcluster)  [unwired: 8 in, 1 out]
        n151 = Merge Errors(w301, w302) -> (w300:errorcluster)
        n152 = call "Remote Communication.vi"("Error In"=w300, "Command"=RT_Command."Update Config") -> ("Error Out"=w294:errorcluster)  [unwired: 4 in, 3 out]
        n153 = call "Set Oscillators.vi"("Error In"=w294) -> ("Error Out"=w292:errorcluster)  [unwired: 1 in, 1 out]
      }
    }
    n154 = case shown="No Error" w9 {
      selector: w9 -> [w14 w16]
      tunnel: [w15 State_Machine."Error"] -> w8
      tunnel: w7 -> [w15 _]
      tunnel: [w14 w16] -> w6
      frame No Error {
      }
      frame Error {
      }
    }
  }
  "Error Out" <- w2
